vi "CAN Log.vi"(6 "Action":enum16{"Update Table", "Clear Table"}(ring), 8 "error in (no error)":errorcluster, 10 "Hexadecimal?":bool=TRUE, 11 "CAN View Table":refnum<vi>) -> (0 "error out":errorcluster, 3 "Output Array":string[][](array[string]))   [LabVIEW 2023, in "HardwareAbstractionLayer_LVOOP.lvlib" / "CAN HAL Lib.lvlib"]
uses:
  CAN HAL Lib.lvlib
  Control/CAN Table.ctl
  Control/CAN Log Data.ctl
  <vilib>/xnet/xnet.llb/XNET Frame CAN.ctl
  <vilib>/xnet/xnet.llb/XNET Frame Type CAN.ctl
  <vilib>/Utility/error.llb/Trim Whitespace One-Sided.vi
panel:
  out "appended array":string[](array[string])
  in  "CAN View Table":T1=-1
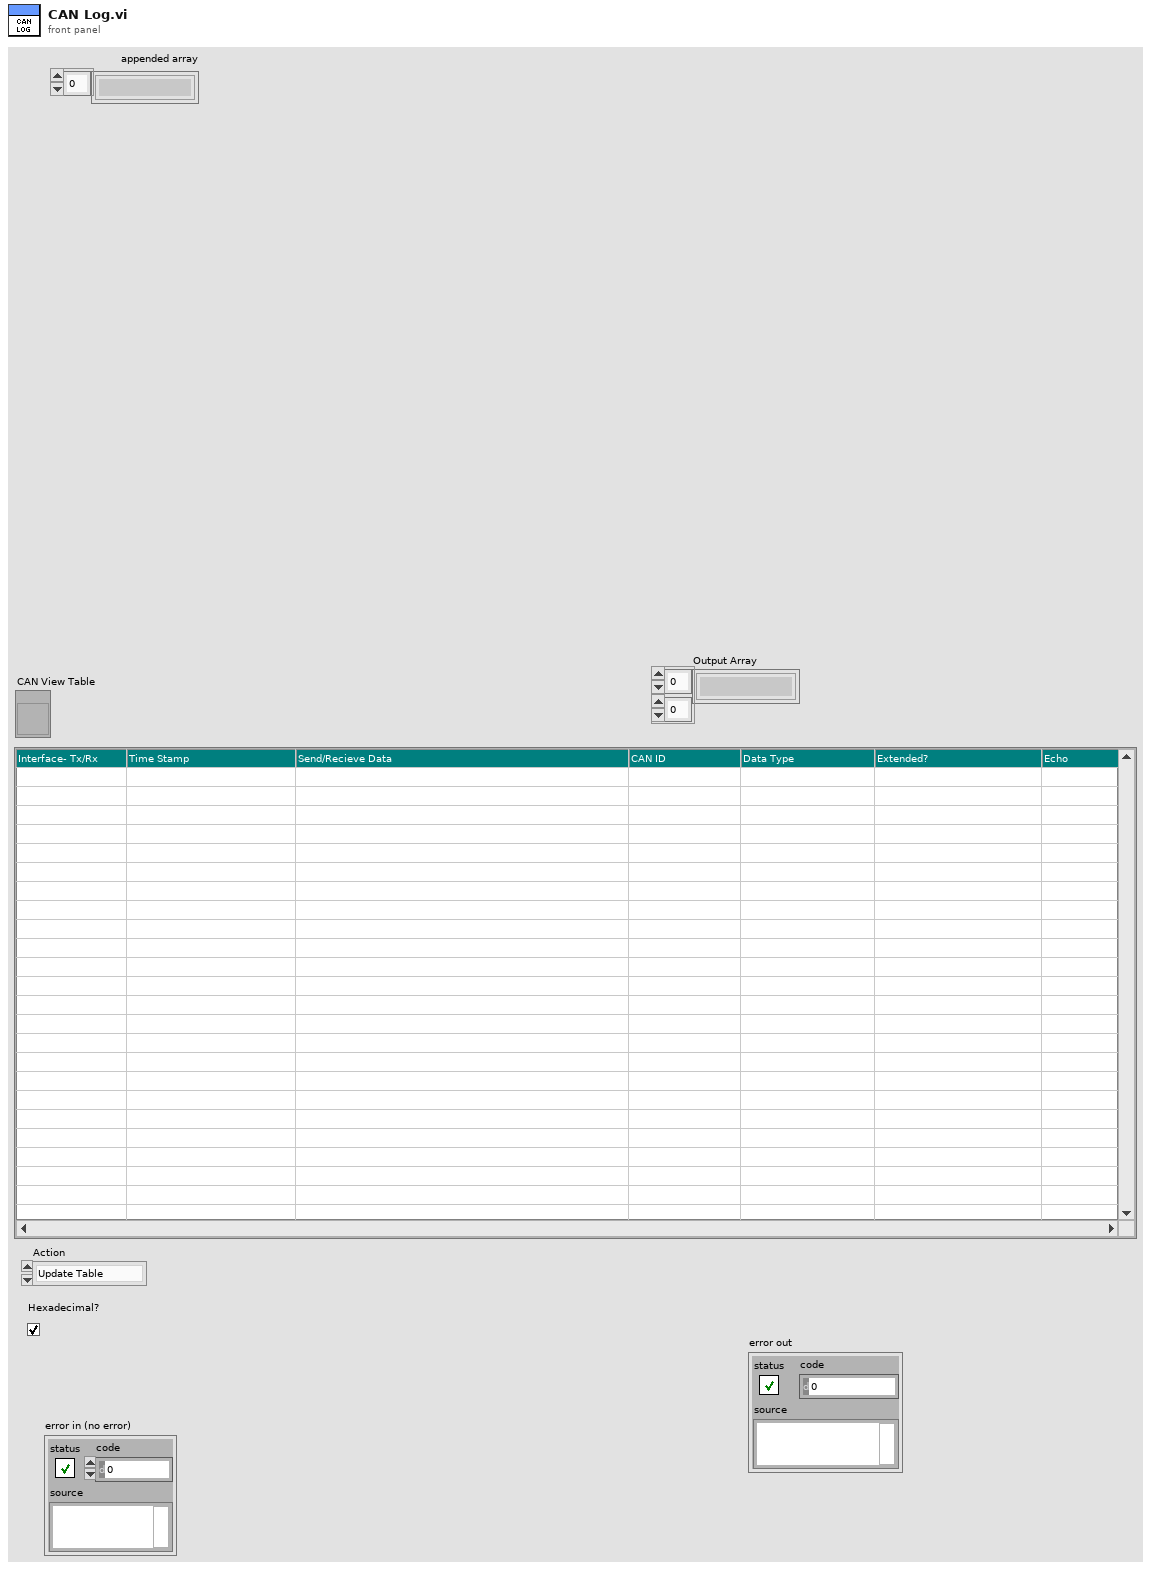
[diagram p1: front panel]
types:
  T1 = typedef "HardwareAbstractionLayer_LVOOP.lvlib/CAN HAL Lib.lvlib/CAN Table.ctl" = i32
  T2 = typedef "HardwareAbstractionLayer_LVOOP.lvlib/CAN HAL Lib.lvlib/CAN Log Data.ctl" = cluster{"Data":T3[], "TX/RX?":enum16{"Tx", "Rx"}, "Interface":string}
  T3 = typedef "XNET Frame CAN.ctl" = cluster{"timestamp":timestamp, "payload":u8[], "identifier":u32, "type":T4, "extended?":bool, "echo?":bool}
  T4 = typedef "XNET Frame Type CAN.ctl" = u8
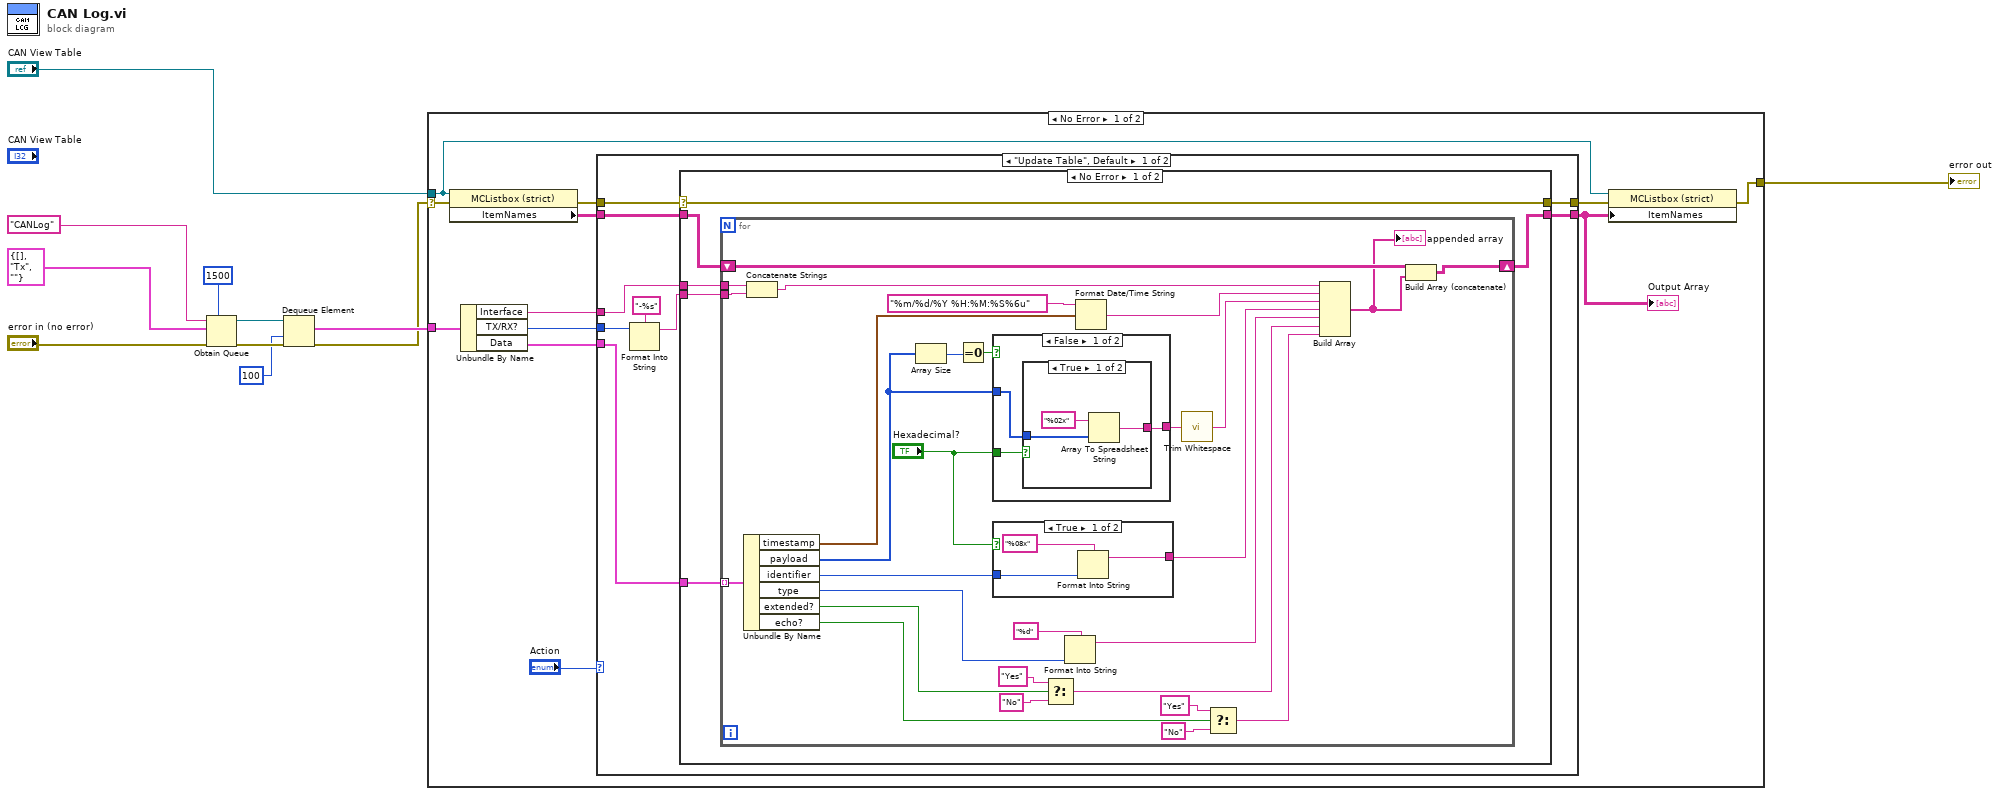
[diagram p0: block diagram]
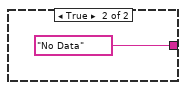
[diagram p3: hidden frame]
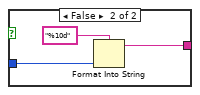
[diagram p4: hidden frame]
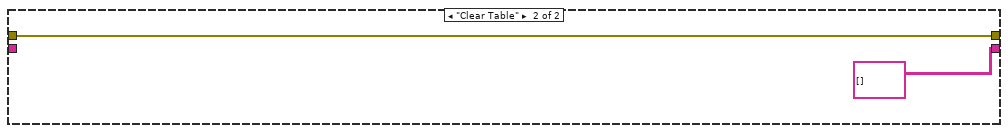
[diagram p6: hidden frame]
diagram:
  n1 = Obtain Queue(max queue size (-1, unlimited)=1500, name (unnamed)="CANLog", element data type=T2 {"Data"=[], "TX/RX?"=enum."Tx", "Interface"=""} ("CAN Data"), error in (no error)="error in (no error)") -> (queue out=w7:refnum<queue>, error out=w6:errorcluster)  [unwired: 1 in, 1 out]
  n2 = Dequeue Element(queue=w7, timeout in ms (-1)=100, error in (no error)=w6) -> (element=w5:T2, error out=w4:errorcluster)  [unwired: 2 out]
  n3 = case shown="No Error" w4 {
    selector: w4 -> [w16 w88]
    tunnel: w5 -> [w19 _]
    tunnel: "CAN View Table" -> [w14 _]
    tunnel: [w12 w88] -> w1
    frame No Error {
      n4 = property class="MCListbox (strict)"(reference=w14, error in=w16) -> (error out=w22:errorcluster, "ItemNames"=w23:string[][])  [unwired: 1 out]
      n5 = Unbundle By Name(w19) -> ("Interface"=w17:string, "TX/RX?"=w15:enum16{"Tx", "Rx"}, "Data"=w18:T3[])
      n6 = case shown="\"Update Table\", Default" "Action" {
        tunnel: w18 -> [w32 _]
        tunnel: w23 -> [w31 _]
        tunnel: [w30 string[][] [] ("Value")] -> w20
        tunnel: [w29 w86] -> w13
        tunnel: w22 -> [w28 w86]
        tunnel: w17 -> [w27 _]
        tunnel: w15 -> [w26 _]
        frame "Update Table", Default {
          n7 = Format Into String(format string="-%s", w26) -> (resulting string=w24:string)  [unwired: 2 in, 1 out]
          n8 = case shown="No Error" w28 {
            selector: w28 -> [w38 w85]
            tunnel: [w38 w85] -> w29
            tunnel: w32 -> [w37 _]
            tunnel: w31 -> [w36 w84]
            tunnel: [w35 w84] -> w30
            tunnel: w27 -> [w34 _]
            tunnel: w24 -> [w33 _]
            frame No Error {
              n9 = for {
                tunnel: w37 -> [w67] mode=indexing
                shift-right: [w60] -> w35
                shift-left: w36 -> [w59]
                tunnel: w34 -> [w53]
                tunnel: w33 -> [w40]
                n10 = Unbundle By Name(w67) -> ("timestamp"=w66:timestamp, "payload"=w55:u8[], "identifier"=w57:u32, "type"=w51:T4, "extended?"=w46:bool, "echo?"=w42:bool)
                n11 = Concatenate Strings(w53, w40) -> (w41:string)
                n12 = Array Size(array=w55) -> (size(s)=w64:i32)
                n13 = Equal To 0?(x=w64) -> (x = 0?=w63:bool)
                n14 = case shown="False" w63 {
                  tunnel: [w68 "No Data"] -> w61
                  tunnel: w55 -> [w70 _]
                  tunnel: "Hexadecimal?" -> [w69 _]
                  frame False {
                    n15 = case shown="True" w69 {
                      tunnel: w70 -> [w72 w75]
                      tunnel: [w71 w74] -> w68
                      frame True {
                        n16 = Array To Spreadsheet String(array=w72, 3:"%02x" ("format string")) -> (spreadsheet string=w71:string)  [unwired: 1 in]
                      }
                      frame False {
                        n17 = Array To Spreadsheet String(array=w75, 3:"%3d" ("format string")) -> (spreadsheet string=w74:string)  [unwired: 1 in]
                      }
                    }
                  }
                  frame True {
                  }
                }
                n18 = case shown="True" "Hexadecimal?" {
                  tunnel: w57 -> [w79 w82]
                  tunnel: [w78 w81] -> w65
                  frame True {
                    n19 = Format Into String(format string="%08x", w79) -> (resulting string=w78:string)  [unwired: 2 in, 1 out]
                  }
                  frame False {
                    n20 = Format Into String(format string="%10d", w82) -> (resulting string=w81:string)  [unwired: 2 in, 1 out]
                  }
                }
                n21 = Select(t="Yes", s=w46, f="No") -> (s? t:f=w47:string)
                n22 = Format Into String(format string="%d", w51) -> (resulting string=w50:string)  [unwired: 2 in, 1 out]
                n23 = Format Date/Time String(time format string (%c)="%m/%d/%Y %H:%M:%S%6u", seconds (now)=w66) -> (date/time string=w56:string)  [unwired: 1 in]
                n24 = call <vilib>:"Trim Whitespace.vi"("string"=w61) -> ("trimmed string"=w58:string)  [unwired: 1 in]
                n25 = Select(t="Yes", s=w42, f="No") -> (s? t:f=w43:string)
                n26 = Build Array(w41, w56, w58, w65, w50, w47, w43) -> (w54:string[])
                "appended array" <- w54
                n27 = Build Array (concatenate)(w59, w54) -> (w60:string[][])
              }
            }
            frame Error {
            }
          }
        }
        frame "Clear Table" {
        }
      }
      "Output Array" <- w20
      n28 = property class="MCListbox (strict)"(reference=w14, error in=w13, "ItemNames"=w20) -> (error out=w12:errorcluster)  [unwired: 1 out]
    }
    frame Error {
    }
  }
  "error out" <- w1
